vi "SelectedTargetToLocation.vi"(9 "Selected Target":i32) -> (0 "Right":bool, 1 "Top":bool, 2 "Left":bool, 3 "Bottom":bool)   [LabVIEW 2011]
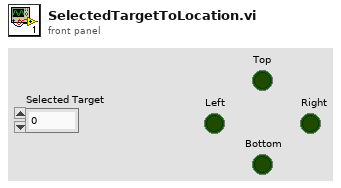
[diagram p1: front panel]
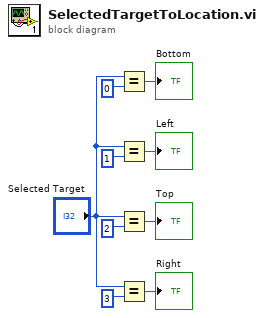
[diagram p0: block diagram]
diagram:
  n1 = Equal?(x="Selected Target", y=0) -> (x = y?=→"Bottom":bool)
  n2 = Equal?(x="Selected Target", y=1) -> (x = y?=→"Left":bool)
  n3 = Equal?(x="Selected Target", y=2) -> (x = y?=→"Top":bool)
  n4 = Equal?(x="Selected Target", y=3) -> (x = y?=→"Right":bool)
